vi "Increment Progress.vi"(11 "Execution UI In":refnum<class "Execution UI.lvclass">) -> (2 "Progress (%)":dbl, 3 "Execution UI Out":refnum<class "Execution UI.lvclass">)   [LabVIEW 2020, in "Execution UI.lvclass"]
uses:
  Execution UI.lvclass
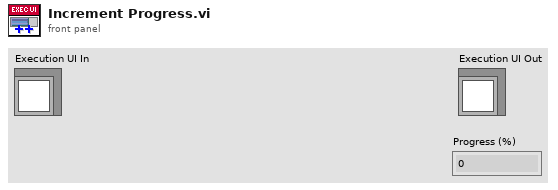
[diagram p1: front panel]
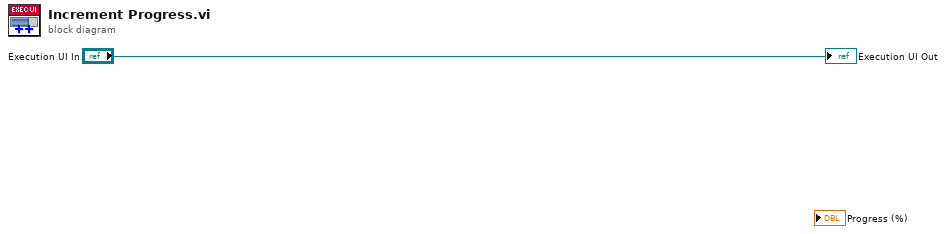
[diagram p0: block diagram]
diagram:
  "Execution UI Out" <- "Execution UI In"
